vi "Joystick Filter.vi"(1 "In":dbl) -> (0 "Out":dbl)   [LabVIEW 2013]
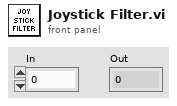
[diagram p1: front panel]
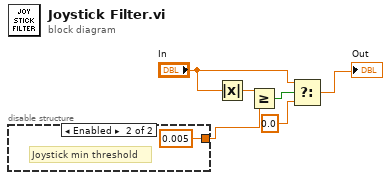
[diagram p0: block diagram]
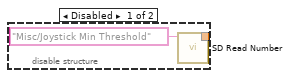
[diagram p2: hidden frame]
diagram:
  n1 = disable-structure shown="Enabled" {
    disable-tunnel: [w8 0.005 ("Numeric")] -> w1
    frame Disabled {
      n2 = call <vilib>:"SD Read Number.vi"("Name"="Misc/Joystick Min Threshold") -> ("Numeric"=w8:dbl)  [unwired: 8 in, 2 out]
    }
    frame Enabled {
      # "Joystick min threshold"
    }
  }
  n3 = Absolute Value(x="In") -> (abs(x)=w2:dbl)
  n4 = Greater Or Equal?(x=w2, y=w1) -> (x >= y?=w3:bool)
  n5 = Select(t="In", s=w3, f=0.0) -> (s? t:f=→"Out":dbl)
